vi "create.vi"   [LabVIEW 2020, in "datasources.lvlib" / "target.lvclass"]
uses:
  target.lvclass
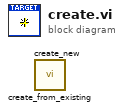
[diagram p0: block diagram]
diagram:
  n1 = call "create_from_existing.vi"() -> ()  [unwired: 11 in, 1 out]
  n2 = call "create_new.vi"() -> ()  [unwired: 11 in, 1 out]
